vi "Yokogawa WT200 Series Measure Mode Value.vi"(0 "VISA resource name":refnum<visa-resource-name>, 11 "error in (no error)":errorcluster) -> (8 "Measure Value":sgl[](array[numeric]) format="%^.3e", 15 "error out":errorcluster)   [LabVIEW 2016]
doc: "This VI configures measurement mode and measures voltage, current and active power for the element 1."
uses:
  Yokogawa WT200 Series.lvlib
panel:
  out "VISA resource name out":refnum<visa-resource-name>
  out "error message":string
  out "error":bool
  # "© 2005 National Instruments.  ALL RIGHTS RESERVED."
  # "WT200 SERIES"
  # "DIGITAL POWER METER"
  # "V1"
  # "A1"
  # "W1"
  # "Wh"
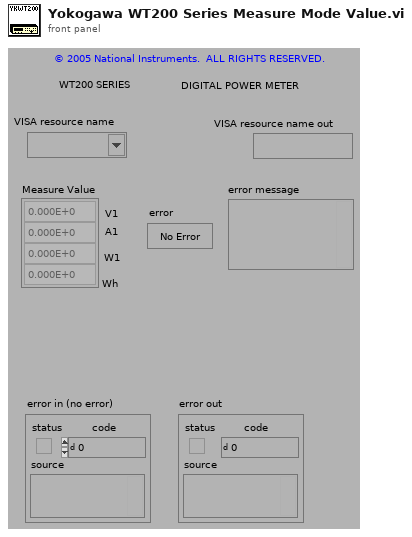
[diagram p1: front panel]
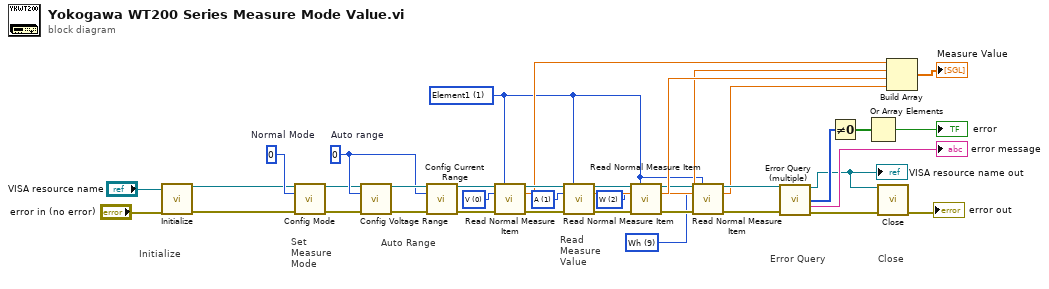
[diagram p0: block diagram]
diagram:
  w5 = u16 9 items=["V", "A", "W", "VA", "var", "PF", "deg", "V Hz", "A Hz", "Wh", "Wh+", "Wh-", "Ah", "Ah+", "Ah-", "Vpk", "Apk", "Math"] ("Measure Item (0: V)")
  w2 = u16 1 items=["", "Element1", "Element2", "Element3", "Sigma"] ("Element (1: Element 1)")
  w20 = u16 0 items=["V", "A", "W", "VA", "var", "PF", "deg", "V Hz", "A Hz", "Wh", "Wh+", "Wh-", "Ah", "Ah+", "Ah-", "Vpk", "Apk", "Math"] ("Measure Item (0: V)")
  w21 = u16 2 items=["V", "A", "W", "VA", "var", "PF", "deg", "V Hz", "A Hz", "Wh", "Wh+", "Wh-", "Ah", "Ah+", "Ah-", "Vpk", "Apk", "Math"] ("Measure Item (0: V)")
  w22 = u16 1 items=["V", "A", "W", "VA", "var", "PF", "deg", "V Hz", "A Hz", "Wh", "Wh+", "Wh-", "Ah", "Ah+", "Ah-", "Vpk", "Apk", "Math"] ("Measure Item (0: V)")
  w34 = u16 0  # Auto range
  w37 = u16 0  # Normal Mode
  # "Error Query"
  # "Close"
  # "Initialize"
  # "Read\nMeasure\nValue"
  # "Auto Range"
  # "Set \nMeasure \nMode"
  n1 = call "Initialize.vi"("VISA resource name"="VISA resource name", "error in (no error)"="error in (no error)") -> ("VISA resource name out"=w17:refnum<visa-resource-name>, "error out"=w16:errorcluster)  [unwired: 11 in, 1 out]
  n2 = call "Config Mode.vi"("VISA resource name"=w17, "Mode (0: RMS)"=w37, "error in (no error)"=w16) -> ("VISA resource name out"=w33:refnum<visa-resource-name>, "error out"=w32:errorcluster)  [unwired: 11 in]
  n3 = call "Config Voltage Range.vi"("VISA resource name"=w33, "V Range (6: 600V)"=w34, "error in (no error)"=w32) -> ("VISA resource name out"=w35:refnum<visa-resource-name>, "error out"=w36:errorcluster)  [unwired: 11 in]
  n4 = call "Config Current Range.vi"("VISA resource name"=w35, "A Range (12: 20A)"=w34, "error in (no error)"=w36) -> ("VISA resource name out"=w30:refnum<visa-resource-name>, "error out"=w31:errorcluster)  [unwired: 11 in]
  n5 = call "Read Normal Measure Item.vi"("VISA resource name"=w30, "Element (1: Element 1)"=w2, "Measure Item (0: V)"=w20, "error in (no error)"=w31) -> ("VISA resource name out"=w27:refnum<visa-resource-name>, "Measure Value"=w23:sgl, "error out"=w29:errorcluster)  [unwired: 9 in]
  n6 = call "Read Normal Measure Item.vi"("VISA resource name"=w27, "Element (1: Element 1)"=w2, "Measure Item (0: V)"=w22, "error in (no error)"=w29) -> ("VISA resource name out"=w26:refnum<visa-resource-name>, "Measure Value"=w24:sgl, "error out"=w28:errorcluster)  [unwired: 9 in]
  n7 = call "Read Normal Measure Item.vi"("VISA resource name"=w26, "Element (1: Element 1)"=w2, "Measure Item (0: V)"=w21, "error in (no error)"=w28) -> ("VISA resource name out"=w4:refnum<visa-resource-name>, "Measure Value"=w25:sgl, "error out"=w7:errorcluster)  [unwired: 9 in]
  n8 = call "Read Normal Measure Item.vi"("VISA resource name"=w4, "Element (1: Element 1)"=w2, "Measure Item (0: V)"=w5, "error in (no error)"=w7) -> ("VISA resource name out"=w3:refnum<visa-resource-name>, "Measure Value"=w1:sgl, "error out"=w6:errorcluster)  [unwired: 9 in]
  n9 = call "Error Query (multiple).vi"("VISA resource name"=w3, "error in (no error)"=w6) -> ("VISA resource name out"=w8:refnum<visa-resource-name>, "Error"=w11:i32[], "Error Message"=→"error message":string, "error out"=w10:errorcluster)  [unwired: 10 in]
  "VISA resource name out" <- w8
  n10 = Not Equal To 0?(x=w11) -> (x != 0?=w12:bool[])
  n11 = Or Array Elements(Boolean array=w12) -> (logical OR=→"error":bool)
  n12 = call "Close.vi"("VISA resource name"=w8, "error in (no error)"=w10) -> ("error out"=→"error out":errorcluster)  [unwired: 13 in]
  n13 = Build Array(w23, w24, w25, w1) -> (→"Measure Value":sgl[])
